vi "Configure Trigger Output.vi"(7 "Enable Manual Trigger Output (F: Disable)":bool, 8 "error in (no error)":errorcluster, 10 "Trigger Output Type (0: Waveform End)":u16(ring) items=["Waveform End", "Position Marker", "Sequence Synchronization", "Burst Done"], 11 "VISA resource name":refnum<visa-resource-name>) -> (0 "error out":errorcluster, 3 "VISA resource name out":refnum<visa-resource-name>)   [LabVIEW 2015, in "Fluke 28x Series.lvlib"]
doc: "Configures the current channel to act as a trigger to another channel by making its output a trigger. \n\n<b>Note</b>: configuring Trigger for use within the same instrument requires a multi-channel instrument, i.e. Fluke 282 or Fluke 284. Trigger can also be configured for use between generators."
uses:
  <instrlib>/Fluke 28x Series/Fluke 28x Series.lvlib
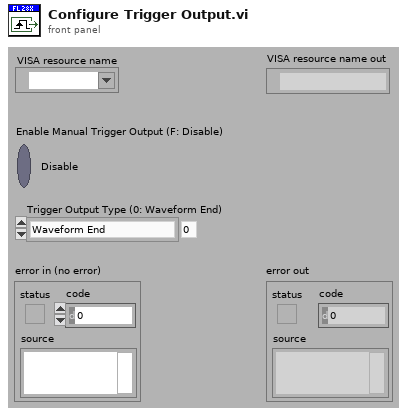
[diagram p1: front panel]
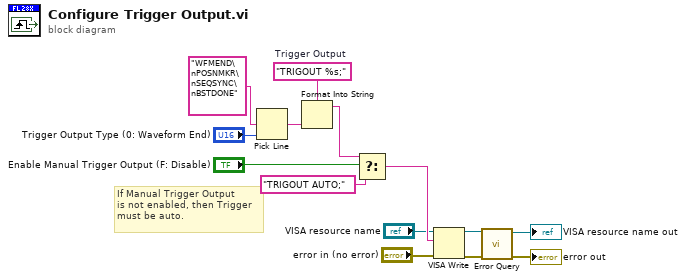
[diagram p0: block diagram]
diagram:
  w12 = "TRIGOUT %s;"  # Trigger Output
  # "If Manual Trigger Output\nis not enabled, then Trigger\nmust be auto."
  n1 = Pick Line(multi-line string="WFMEND\nPOSNMKR\nSEQSYNC\nBSTDONE", line index="Trigger Output Type (0: Waveform End)") -> (output string=w11:string)  [unwired: 1 in]
  n2 = Format Into String(format string=w12, w11) -> (resulting string=w8:string)  [unwired: 2 in, 1 out]
  n3 = Select(t=w8, s="Enable Manual Trigger Output (F: Disable)", f="TRIGOUT AUTO;") -> (s? t:f=w7:string)
  n4 = VISA Write(VISA resource name="VISA resource name", write buffer=w7, error in (no error)="error in (no error)") -> (VISA resource name out=w5:refnum<visa-resource-name>, error out=w4:errorcluster)  [unwired: 1 out]
  n5 = call <instrlib>:"Error Query.vi"("error in (no error)"=w4, "VISA resource name"=w5) -> ("error out"=→"error out":errorcluster, "VISA resource name out"=→"VISA resource name out":refnum<visa-resource-name>)  [unwired: 6 in, 2 out]
